vi "test Error Wrapping - No Execute On Error In.vi"(8 "error in (no error)":errorcluster, 11 "TestCase in":refnum<class "Error Tests.lvclass">) -> (0 "error out":errorcluster, 3 "TestCase out":refnum<class "Error Tests.lvclass">)   [LabVIEW 2020, in "Error Tests.lvclass"]
uses:
  Error Tests.lvclass
  <vilib>/Utility/file.llb/Application Directory.vi
  <vilib>/Utility/libraryn.llb/Check if File or Folder Exists.vi
  <vilib>/addons/_JKI Toolkits/VI Tester/TestCase.llb/TestCase.lvclass
  C:/Program Files/National Instruments/LabVIEW 2024/vi.lib/addons/_JKI Toolkits/VI Tester/TestCase.llb/TestCase.lvclass
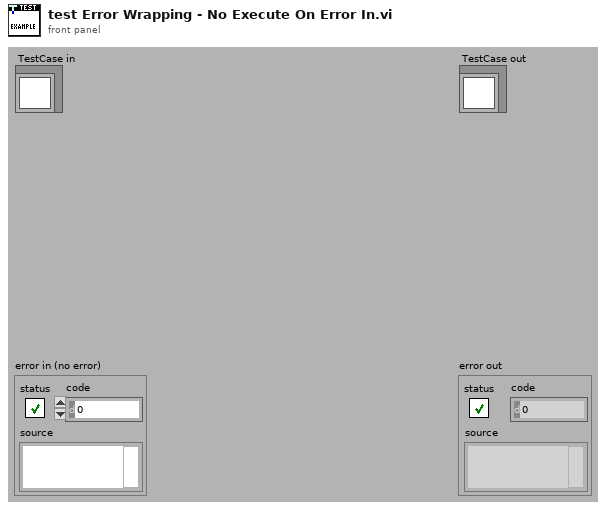
[diagram p1: front panel]
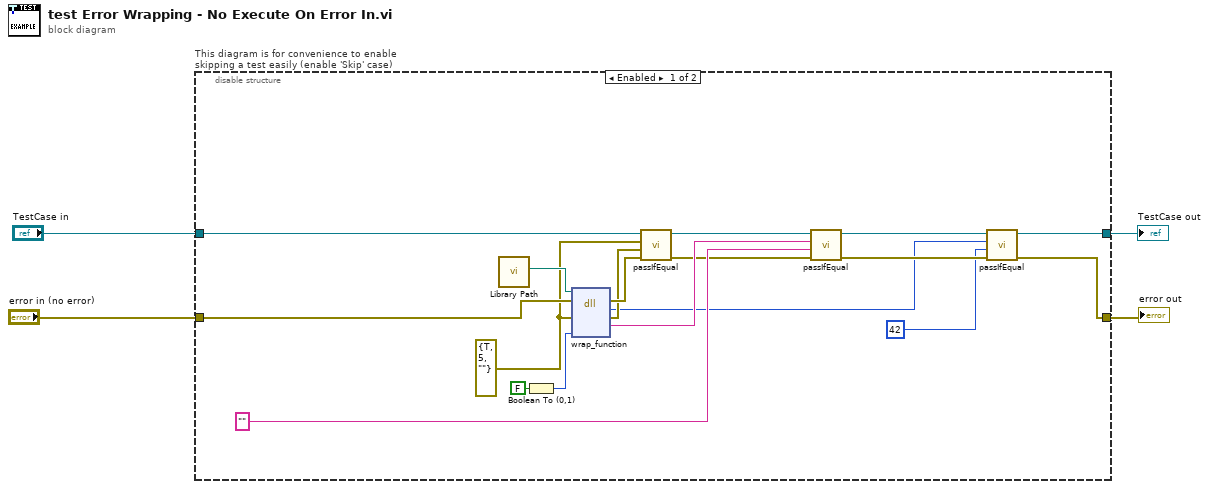
[diagram p0: block diagram]
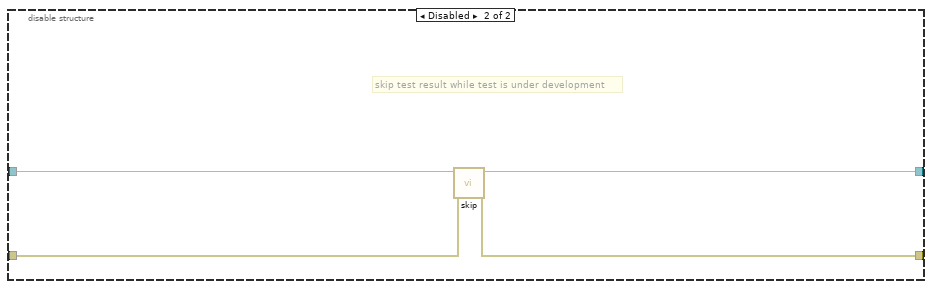
[diagram p2: hidden frame]
diagram:
  n1 = disable-structure "This diagram is for convenience to enable skipping a test easily (enable 'Skip' case)" shown="Enabled" {
    disable-tunnel: "TestCase in" -> [w15 w26]
    disable-tunnel: [w9 w24] -> w1
    disable-tunnel: [w11 w25] -> w3
    disable-tunnel: "error in (no error)" -> [w17 w23]
    frame Enabled {
      w13 = errorcluster {"status"=TRUE, "code"=5, "source"=""} ("error in (no error)")
      n2 = call "Library Path.vi"() -> ("Library Path"=w22:path)  [unwired: 11 in]
      n3 = Boolean To (0,1)(Boolean=FALSE) -> (0, 1=w5:i16)
      n4 = dll-call lib="C:/Users/JamesMcNally/Documents/RustInterop/Rust-LabVIEW-Interop/target/debug/labview_test_library.dll" fn="wrap_function"(path in=w22, error in=w17, "code"=w13, "create_eror"=w5) -> (error out=w20:errorcluster, "return type"=w8:i32, "code"=w12:errorcluster, "text"=w19:string)  [unwired: 3 in, 1 out]
      n5 = call-dynamic "passIfEqual.vi"("error in (no error)"=w20, "y"=w12, "x"=w13, "TestCase in"=w15) -> ("error out"=w16:errorcluster, "TestCase out"=w14:refnum<class "Error Tests.lvclass">)  [unwired: 6 in]
      n6 = call-dynamic "passIfEqual.vi"("error in (no error)"=w16, "y"="", "x"=w19, "TestCase in"=w14) -> ("error out"=w21:errorcluster, "TestCase out"=w10:refnum<class "Error Tests.lvclass">)  [unwired: 6 in]
      n7 = call-dynamic "passIfEqual.vi"("error in (no error)"=w21, "y"=42 ("return type"), "x"=w8, "TestCase in"=w10) -> ("error out"=w11:errorcluster, "TestCase out"=w9:refnum<class "Error Tests.lvclass">)  [unwired: 6 in]
    }
    frame Disabled {
      # "skip test result while test is under development"
      n8 = call <vilib>:"skip.vi"("error in (no error)"=w23, "TestCase in"=w26) -> ("error out"=w25:errorcluster, "TestCase out"=w24:refnum<class "Error Tests.lvclass">)  [unwired: 8 in]
    }
  }
  "error out" <- w3
  "TestCase out" <- w1
